vi "No Inline Plugins.vi"(8 "error in (no error)":errorcluster, 11 "Framework in":refnum<class "Framework.lvclass">) -> (0 "error out":errorcluster, 2 "no inline?":bool, 3 "Framework out":refnum<class "Framework.lvclass">)   [LabVIEW 2017, in "DSF Core.lvlib" / "Framework.lvclass"]
uses:
  Framework.lvclass
  Framework.lvclass/Framework.ctl
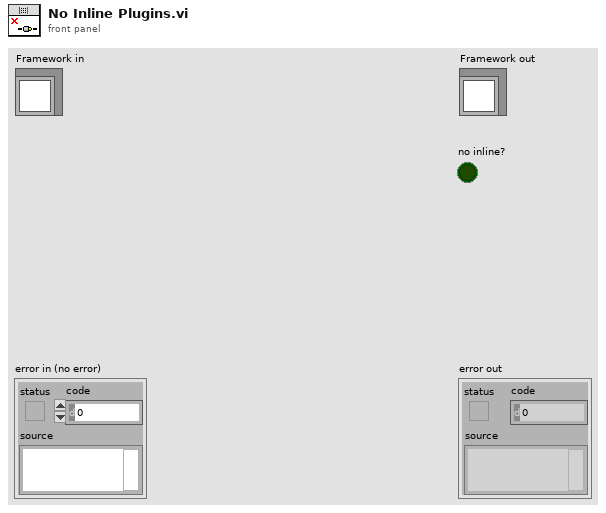
[diagram p1: front panel]
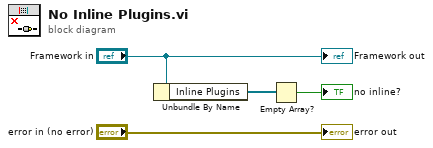
[diagram p0: block diagram]
diagram:
  n1 = Unbundle By Name("Framework in") -> ("Inline Plugins"=w2:refnum<class "Plugin.lvclass">[])
  n2 = Empty Array?(array=w2) -> (empty?=→"no inline?":bool)
  "error out" <- "error in (no error)"
  "Framework out" <- "Framework in"
